vi "Read_filename.vi"(8 "error in":errorcluster, 11 "Filename (ini)":string="Config_Ver_2\\state_library") -> (0 "error out":errorcluster, 3 "Strings []":string[](array[string]))   [LabVIEW 2021]
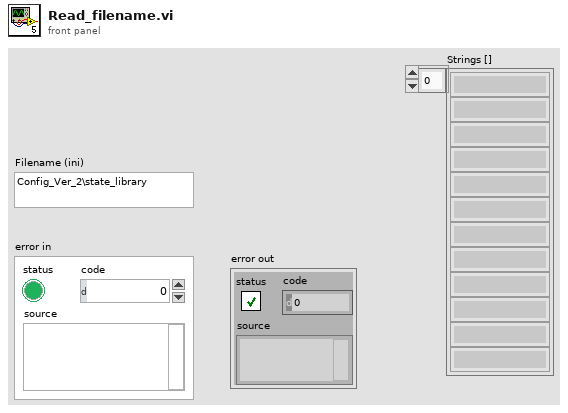
[diagram p1: front panel]
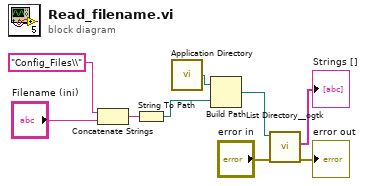
[diagram p0: block diagram]
diagram:
  n1 = Concatenate Strings("Config_Files\\" ("string"), "Filename (ini)") -> (w3:string)
  n2 = String To Path(string=w3) -> (path=w4:path)
  n3 = call <vilib>:"Application Directory.vi"() -> ("Application Directory"=w6:path)
  n4 = Build Path(base path=w6, name or relative path=w4) -> (appended path=w2:path)
  n5 = call <userlib>:"List Directory__ogtk.vi"("error in (no error)"="error in", "directory path"=w2) -> ("error out"=→"error out":errorcluster, "file names"=→"Strings []":string[])  [unwired: 2 in, 2 out]
